vi "8. CoffeeMaker Store and Read Data.vi"() -> ()   [LabVIEW 2018]
doc: "Coffee Machine Version 1.0: store and read non-volatile data of coffee units and brewing chamber operations"
uses:
  Controls/States.ctl
  <vilib>/Utility/miscctls.llb/LVMinMaxIncTypeDef.ctl
  <vilib>/Utility/file.llb/Read Delimited Spreadsheet (DBL).vi
  <vilib>/Utility/file.llb/Read Delimited Spreadsheet (string).vi
  <vilib>/Utility/file.llb/Write Delimited Spreadsheet (DBL).vi
panel:
  out "s? t:f":enum16{"next state", "current state"}(ring)
  out "error out":errorcluster
  in  "error in (no error)":errorcluster
  in  "Power Switch":bool
  in  "Simulation":cluster{"Water":dbl, "Coffee":dbl, "Milk":dbl} caption="Wasser" {"Milk" scale=0.0..100.0; "Water" scale=0.0..100.0; "Coffee" scale=0.0..100.0}
  out "Display":T1 {"Coffee" scale=0.0..80.0; "Brewing Chamber" scale=0.0..80.0}
  in  "Coffee Selection":T2 caption="Selection" {"Type" min=0 max=2 step=1 scale=0.0..2.0}
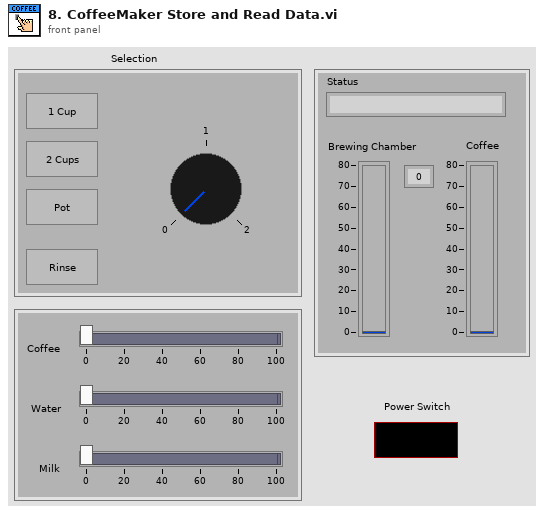
[diagram p1: front panel]
types:
  T1 = cluster{"Brewing Chamber":dbl, "Coffee":dbl, "Status":string, "Remaining Time:":i32}
  T2 = cluster{"1 Cup":bool, "2 Cups":bool, "Pot":bool, "Rinse":bool, "Type":i8}
  T3 = cluster{"Status":refnum<vi>, "Brewing Chamber":refnum<vi>, "Coffee":refnum<vi>, "Power Switch":refnum<vi>}
  T4 = enum8{"Enabled", "Disabled", "Disabled and Grayed Out"}
  T5 = typedef "LVMinMaxIncTypeDef.ctl" = cluster{"Minimum":dbl, "Maximum":dbl, "Increment":dbl}
  T6 = typedef "States.ctl" = enum16{"Initialize", "Set Language", "Wait for Power On", "Heat up", "Check and Wait for Water", "Rinsing", "Check Resources", "User Input", "Grinding", "Boiling", "Pouring", "Rinse before Stop", "Write Data", "Stop"}
  T7 = cluster{"Coffee":refnum<vi>, "Water":refnum<vi>, "Milk":refnum<vi>}
  T8 = cluster{"Coffee Selection":refnum<vi>, "1 Cup":refnum<vi>, "2 Cups":refnum<vi>, "Pot":refnum<vi>, "Rinse":refnum<vi>, "Type":refnum<vi>}
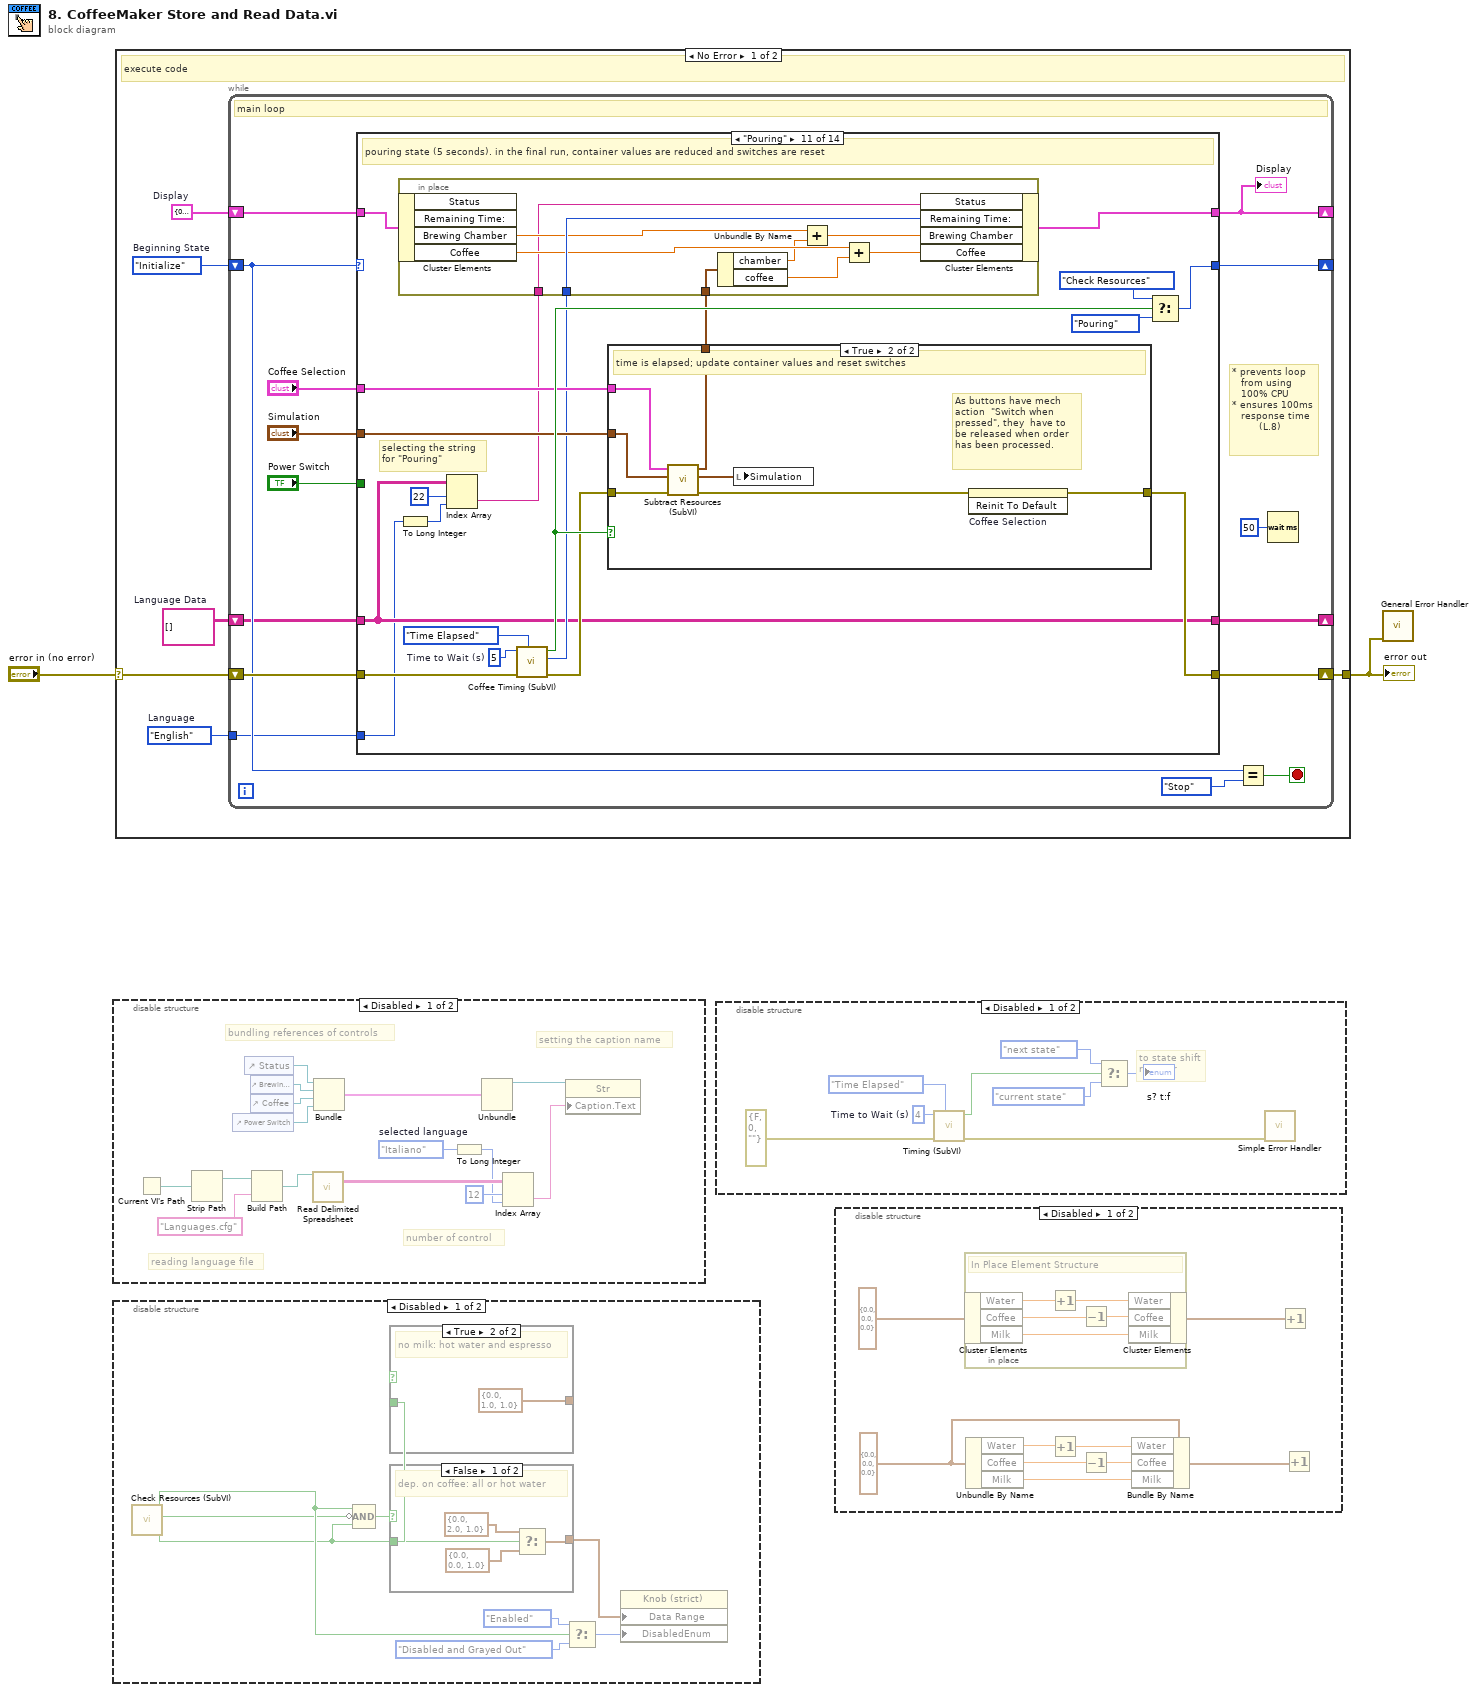
[diagram p0: block diagram]
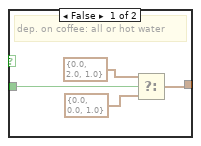
[diagram p3: hidden frame]
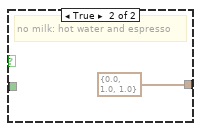
[diagram p4: hidden frame]
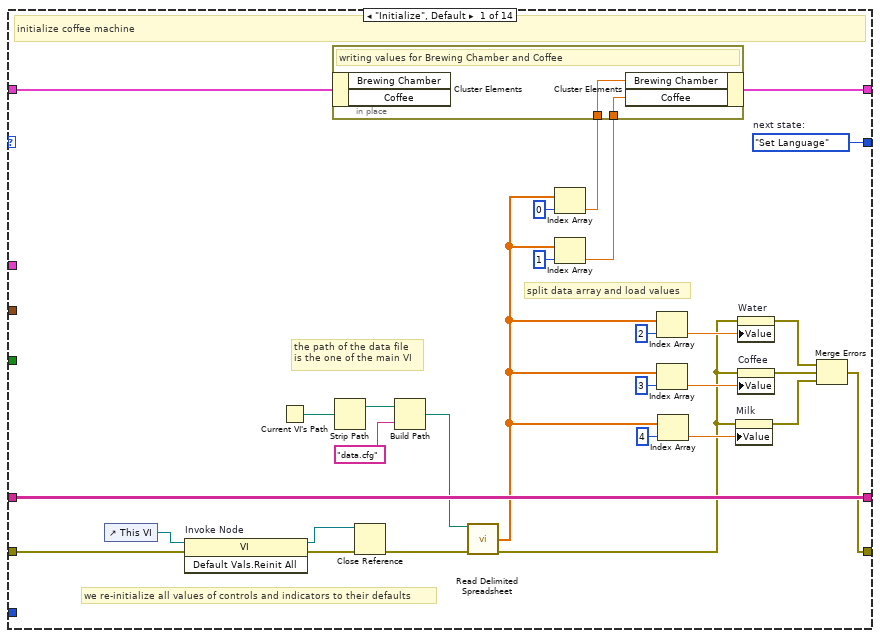
[diagram p8: hidden frame]
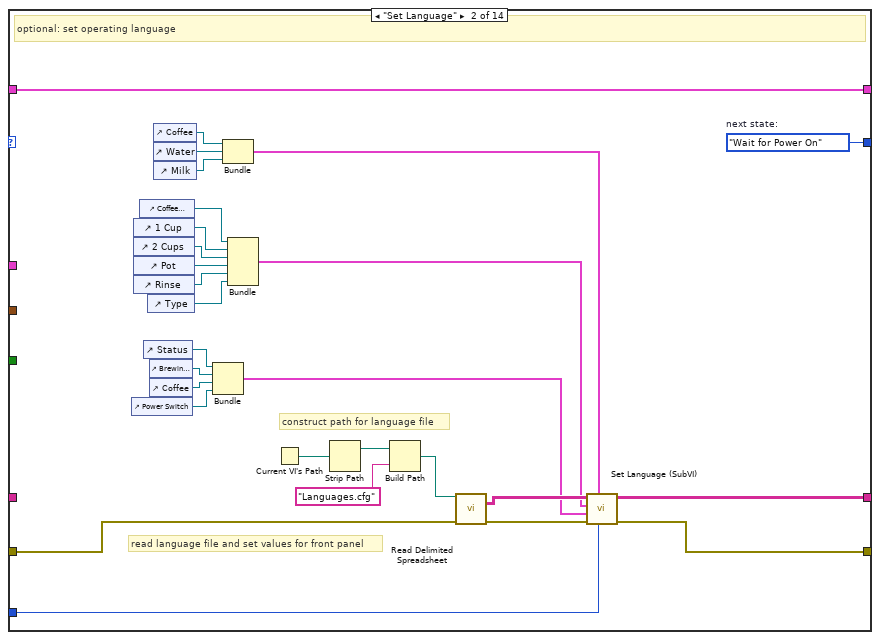
[diagram p9: hidden frame]
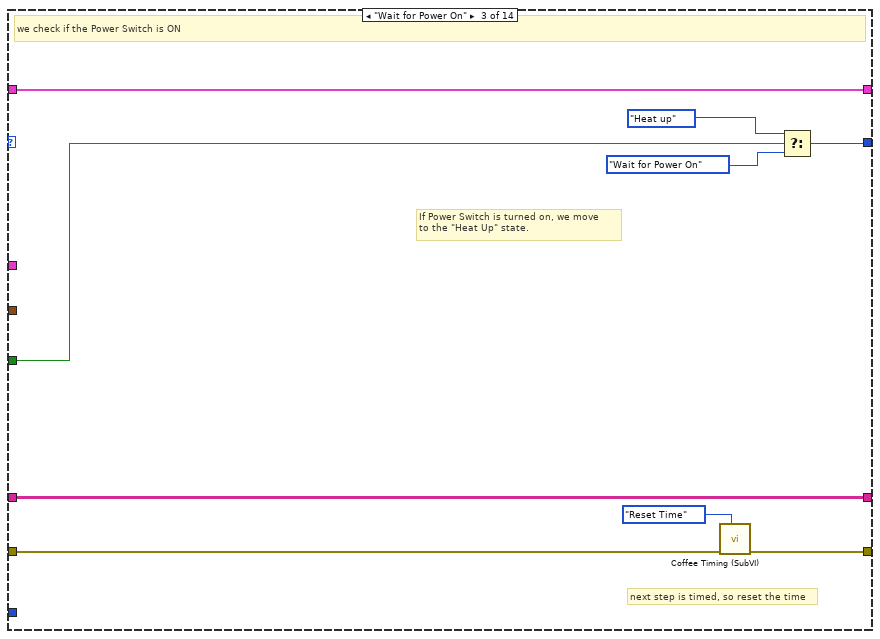
[diagram p10: hidden frame]
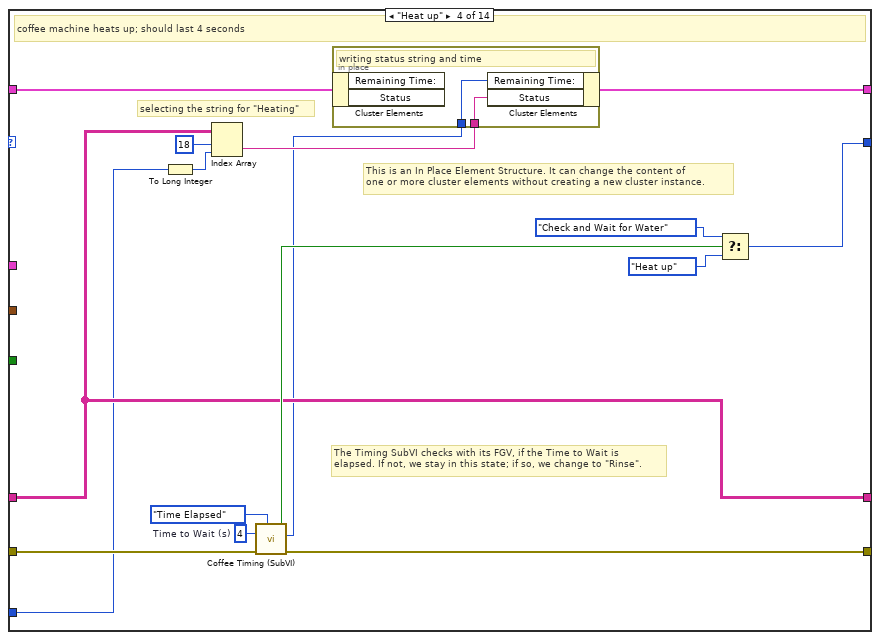
[diagram p11: hidden frame]
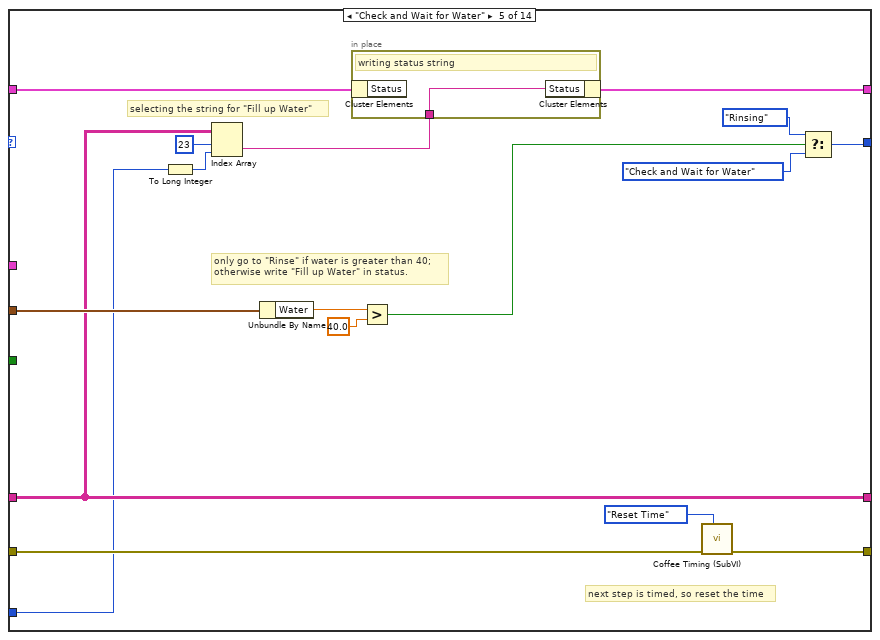
[diagram p12: hidden frame]
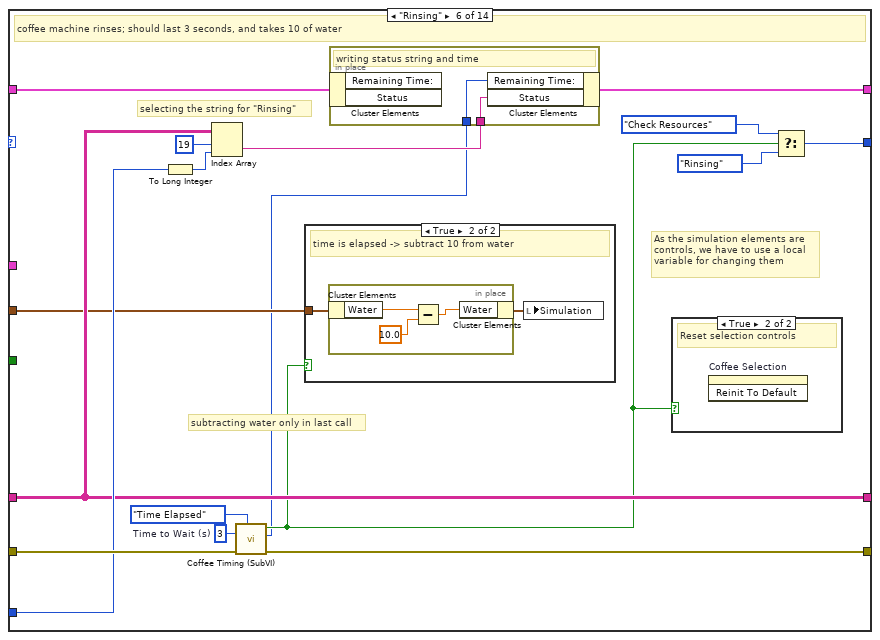
[diagram p13: hidden frame]
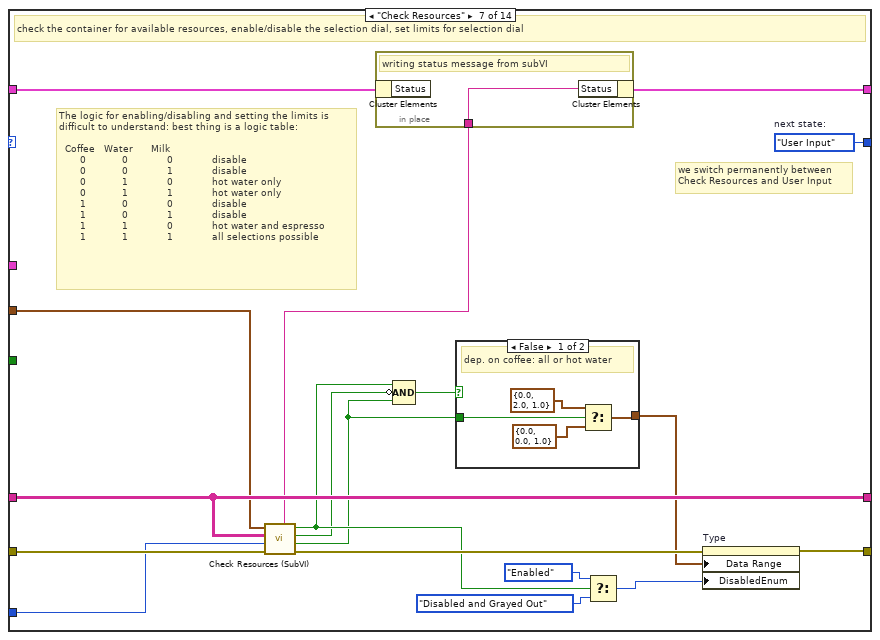
[diagram p16: hidden frame]
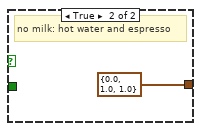
[diagram p17: hidden frame]
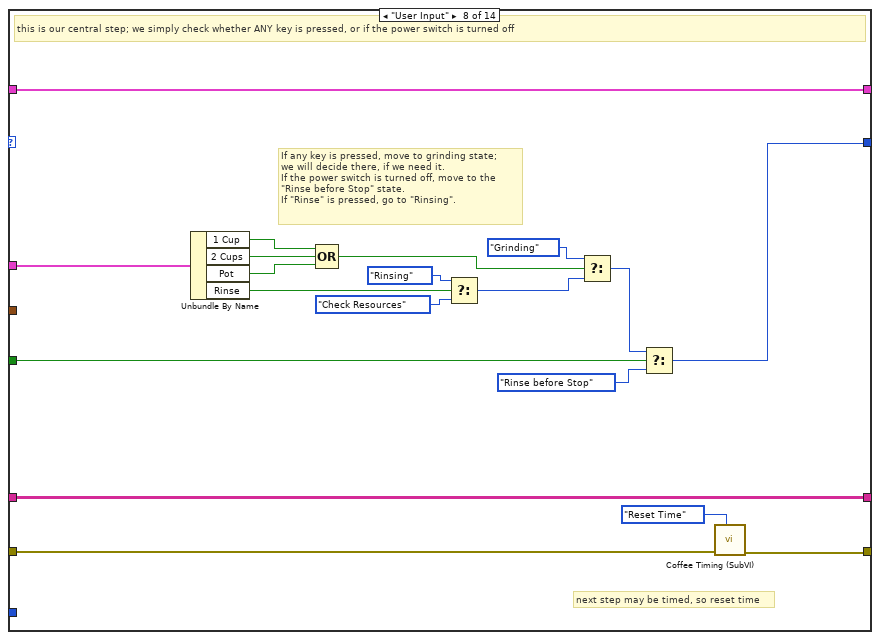
[diagram p18: hidden frame]
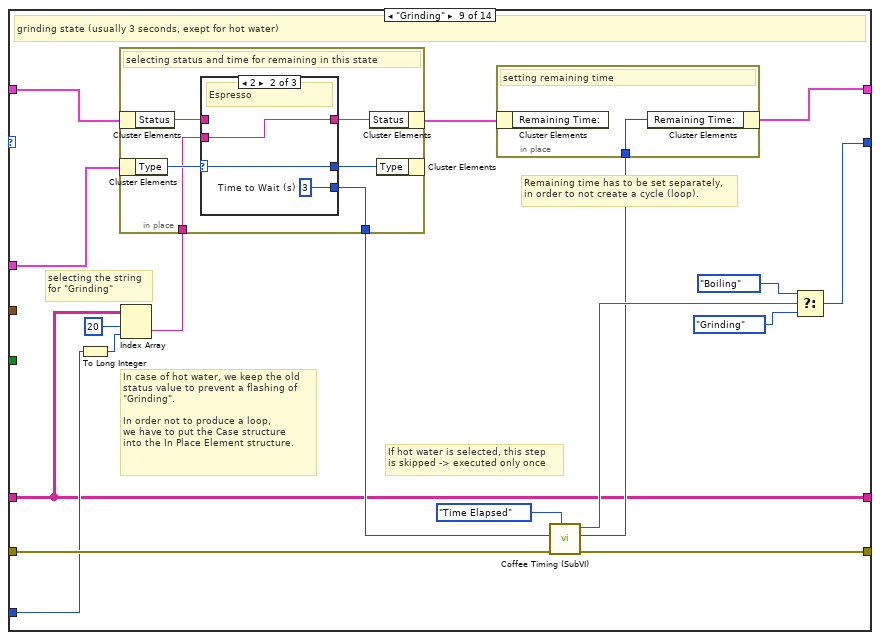
[diagram p19: hidden frame]
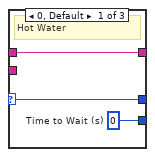
[diagram p20: hidden frame]
diagram:
  n1 = disable-structure shown="Disabled" {
    frame Disabled {
      w5 = enum16{"English", "Deutsch", "Italiano"}."Italiano"  # selected language
      # "setting the caption name"
      # "number of control"
      # "reading language file"
      # "bundling references of controls"
      n2 = Current VI's Path() -> (path=w11:path)
      n3 = Strip Path(path=w11) -> (stripped path=w10:path)  [unwired: 1 out]
      n4 = control-ref of="Power Switch"() -> (w17:refnum<vi>)
      n5 = control-ref of="Status"() -> (w14:refnum<vi>)
      n6 = control-ref of="Brewing Chamber"() -> (w15:refnum<vi>)
      n7 = control-ref of="Coffee"() -> (w16:refnum<vi>)
      n8 = Build Path(base path=w10, name or relative path="Languages.cfg") -> (appended path=w8:path)
      n9 = call-poly <vilib>:"Read Delimited Spreadsheet.vi"("file path (dialog if empty)"=w8) -> ("all rows"=w7:string[][])  [unwired: 9 in, 5 out]
      n10 = Bundle("Status"=w14, "Brewing Chamber"=w15, "Coffee"=w16, "Power Switch"=w17) -> (w13:T3)  [unwired: 1 in]
      n11 = To Long Integer(number=w5) -> (32bit integer=w4:i32)
      n12 = Unbundle(w13) -> ("Status"=w12:refnum<vi>)  [unwired: 3 out]
      n13 = Index Array(array=w7, index (row)=12, index (col)=w4) -> (element=w3:string)
      n14 = property class="Str"(reference=w12, "Caption.Text"=w3) -> ()  [unwired: 1 in, 2 out]
    }
    frame Enabled {
    }
  }
  n15 = disable-structure shown="Disabled" {
    frame Disabled {
      n16 = call "Check Resources (SubVI).vi"() -> ("Coffee ok?"=w18:bool, "Milk ok?"=w19:bool, "Water ok?"=w20:bool)  [unwired: 7 in, 2 out]
      n17 = Compound Arithmetic op=AND(w20, invert w19, w18) -> (w22:bool)
      n18 = case shown="True" {
        selector: _ -> [_ _]
        tunnel: w18 -> [w27 _]
        tunnel: [w26 T5 {"Minimum"=0.0, "Maximum"=1.0, "Increment"=1.0} ("Data Entry Limits")] -> _
        frame False {
          # "dep. on coffee: all or hot water"
          n19 = Select(t=T5 {"Minimum"=0.0, "Maximum"=2.0, "Increment"=1.0} ("Data Entry Limits"), s=w27, f=T5 {"Minimum"=0.0, "Maximum"=0.0, "Increment"=1.0} ("Data Entry Limits")) -> (s? t:f=w26:T5)
        }
        frame True {
          # "no milk: hot water and espresso"
        }
      }
      n20 = case shown="False" w22 {
        tunnel: w18 -> [w32 _]
        tunnel: [w31 T5 {"Minimum"=0.0, "Maximum"=1.0, "Increment"=1.0} ("Data Entry Limits")] -> w21
        frame False {
          # "dep. on coffee: all or hot water"
          n21 = Select(t=T5 {"Minimum"=0.0, "Maximum"=2.0, "Increment"=1.0} ("Data Entry Limits"), s=w32, f=T5 {"Minimum"=0.0, "Maximum"=0.0, "Increment"=1.0} ("Data Entry Limits")) -> (s? t:f=w31:T5)
        }
        frame True {
          # "no milk: hot water and espresso"
        }
      }
      n22 = Select(t=T4."Enabled" ("Disabled"), s=w20, f=T4."Disabled and Grayed Out" ("Disabled")) -> (s? t:f=w23:T4)
      n23 = property on="Property Node" class="Knob (strict)"("Data Range"=w21, "DisabledEnum"=w23) -> ()  [unwired: 2 in, 2 out]
    }
    frame Enabled {
    }
  }
  n24 = case shown="No Error" "error in (no error)" {
    selector: "error in (no error)" -> [w40 w365]
    tunnel: [w41 w365] -> w1
    frame No Error {
      w36 = T1 {"Brewing Chamber"=0.0, "Coffee"=0.0, "Status"="", "Remaining Time:"=0}  # Display
      w37 = enum16{"English", "Deutsch", "Italiano"}."English"  # Language
      w38 = string[][] []  # Language Data
      w39 = States."Initialize"  # Beginning State
      # "execute code"
      n25 = while {
        shift-right: [w53] -> _
        shift-left: w39 -> [w52]
        shift-right: [w46] -> _
        shift-left: w38 -> [w45]
        shift-right: [w42] -> _
        shift-left: w36 -> [w49]
        shift-right: [w56] -> w41
        shift-left: w40 -> [w55]
        tunnel: w37 -> [w43]
        stop <- w50 stop-if-true
        # "* prevents loop\n   from using\n   100% CPU\n* ensures 100ms\n   response time\n         (L.8)"
        # "main loop"
        n26 = case shown="\"Pouring\"" w52 {
          tunnel: [w74 w108 w119 w139 w150 w176 w192 w225 w243 w274 w287 w334 w353 w361] -> w56
          tunnel: w55 -> [w85 w109 w120 w140 w151 w177 w202 w226 w244 w275 w297 w335 w354 w361]
          tunnel: "Power Switch" -> [_ _ w124 _ _ _ _ w223 _ _ _ _ _ _]
          tunnel: [w84 w106 w123 w136 w157 w173 w196 w222 w240 w270 w294 w331 States."Stop" ("f") States."Stop" ("f")] -> w53
          tunnel: [w63 w105 w117 w131 w143 w169 w197 w213 w233 w276 w298 w328 w351 w363] -> w42
          tunnel: w49 -> [w64 w105 w117 w132 w149 w170 w199 w213 w245 w277 w299 w329 w351 w363]
          tunnel: "Coffee Selection" -> [_ _ _ _ _ _ _ w221 w237 _ w289 _ _ _]
          tunnel: "Simulation" -> [_ _ _ _ w156 w163 w200 _ _ _ w290 w323 w352 _]
          tunnel: [w83 w107 w116 w130 w146 w165 w201 w227 w229 w264 w282 w324 w359 w362] -> w46
          tunnel: w45 -> [w83 _ w116 w130 w146 w165 w201 w227 w229 w264 w282 w324 w359 w362]
          tunnel: w43 -> [_ w92 _ w127 w145 w166 w185 _ w230 w263 w281 w325 _ _]
          frame "Initialize", Default {
            w84 = States."Set Language"  # next state:
            # "split data array and load values"
            # "the path of the data file \nis the one of the main VI"
            # "we re-initialize all values of controls and indicators to their defaults"
            # "initialize coffee machine"
            n27 = control-ref of="This VI"() -> (w59:refnum<vi>)
            n28 = invoke on="Invoke Node" class="VI" method="Default Vals.Reinit All"(reference=w59, error in=w85) -> (reference out=w58:refnum<vi>, error out=w57:errorcluster)  [unwired: 1 in, 1 out]
            n29 = Current VI's Path() -> (path=w81:path)
            n30 = Strip Path(path=w81) -> (stripped path=w80:path)  [unwired: 1 out]
            n31 = Close Reference(reference=w58, error in (no error)=w57) -> (error out=w82:errorcluster)
            n32 = Build Path(base path=w80, name or relative path="data.cfg") -> (appended path=w78:path)
            n33 = call-poly <vilib>:"Read Delimited Spreadsheet.vi"("file path (dialog if empty)"=w78, "error in (no error)"=w82) -> ("first row"=w77:dbl[], "error out"=w60:errorcluster)  [unwired: 8 in, 4 out]
            n34 = Index Array "Index Array"(array=w77, index=0) -> (element=w62:dbl)
            n35 = Index Array(array=w77, index=1) -> (element=w61:dbl)
            n36 = in-place {
              in-place-border: w62 -> [w87]
              in-place-border: w61 -> [w86]
              # "writing values for Brewing Chamber and Coffee"
              n37 = in-place-cluster #1(w64) -> ()  [unwired: 2 out]
              n38 = in-place-cluster #1("Brewing Chamber"=w87, "Coffee"=w86) -> (w63:T1)
            }
            n39 = Index Array(array=w77, index=2) -> (element=w68:dbl)
            n40 = Index Array(array=w77, index=3) -> (element=w66:dbl)
            n41 = Index Array(array=w77, index=4) -> (element=w76:dbl)
            n42 = property on="Milk" class="Slide (strict)"(error in=w60, "Value"=w76) -> (error out=w75:errorcluster)  [unwired: 1 in, 1 out]
            n43 = property on="Water" class="Slide (strict)"(error in=w60, "Value"=w68) -> (error out=w67:errorcluster)  [unwired: 1 in, 1 out]
            n44 = property on="Coffee" class="Slide (strict)"(error in=w60, "Value"=w66) -> (error out=w65:errorcluster)  [unwired: 1 in, 1 out]
            n45 = Merge Errors(w67, w65, w75) -> (w74:errorcluster)
          }
          frame "Set Language" {
            w106 = States."Wait for Power On"  # next state:
            # "construct path for language file"
            # "read language file and set values for front panel"
            # "optional: set operating language"
            n46 = control-ref of="Power Switch"() -> (w95:refnum<vi>)
            n47 = control-ref of="1 Cup"() -> (w103:refnum<vi>)
            n48 = control-ref of="2 Cups"() -> (w102:refnum<vi>)
            n49 = control-ref of="Pot"() -> (w101:refnum<vi>)
            n50 = control-ref of="Rinse"() -> (w100:refnum<vi>)
            n51 = control-ref of="Coffee Selection"() -> (w104:refnum<vi>)
            n52 = control-ref of="Status"() -> (w98:refnum<vi>)
            n53 = control-ref of="Type"() -> (w99:refnum<vi>)
            n54 = control-ref of="Brewing Chamber"() -> (w97:refnum<vi>)
            n55 = control-ref of="Coffee"() -> (w96:refnum<vi>)
            n56 = control-ref of="Coffee"() -> (w91:refnum<vi>)
            n57 = control-ref of="Water"() -> (w90:refnum<vi>)
            n58 = control-ref of="Milk"() -> (w89:refnum<vi>)
            n59 = Bundle("Status"=w98, "Brewing Chamber"=w97, "Coffee"=w96, "Power Switch"=w95) -> (w93:T3)  [unwired: 1 in]
            n60 = Bundle("Coffee"=w91, "Water"=w90, "Milk"=w89) -> (w88:T7)  [unwired: 1 in]
            n61 = Bundle("Coffee Selection"=w104, "1 Cup"=w103, "2 Cups"=w102, "Pot"=w101, "Rinse"=w100, "Type"=w99) -> (w94:T8)  [unwired: 1 in]
            n62 = Current VI's Path() -> (path=w110:path)
            n63 = Strip Path(path=w110) -> (stripped path=w111:path)  [unwired: 1 out]
            n64 = Build Path(base path=w111, name or relative path="Languages.cfg") -> (appended path=w113:path)
            n65 = call-poly <vilib>:"Read Delimited Spreadsheet.vi"("file path (dialog if empty)"=w113, "error in (no error)"=w109) -> ("all rows"=w115:string[][], "error out"=w114:errorcluster)  [unwired: 8 in, 4 out]
            n66 = call "Set Language (SubVI).vi"("Language (English)"=w92, "Simulation \nReferences"=w88, "error in (no error)"=w114, "Status\nReferences"=w93, "Selection \nReferences"=w94, "Language Data"=w115) -> ("error out"=w108:errorcluster, "Language Data Out"=w107:string[][])  [unwired: 4 in]
          }
          frame "Wait for Power On" {
            # "next step is timed, so reset the time"
            # "If Power Switch is turned on, we move\nto the \"Heat Up\" state."
            # "we check if the Power Switch is ON"
            n67 = call "Coffee Timing (SubVI).vi"("Function"=enum16{"Reset Time", "Time Elapsed"}."Reset Time", "error in (no error)"=w120) -> ("error out"=w119:errorcluster)  [unwired: 7 in, 2 out]
            n68 = Select(t=States."Heat up" ("Beginning State"), s=w124, f=States."Wait for Power On") -> (s? t:f=w123:T6)
          }
          frame "Heat up" {
            w137 = 4  # Time to Wait (s)
            # "selecting the string for \"Heating\""
            # "This is an In Place Element Structure. It can change the content of\none or more cluster elements without creating a new cluster instance."
            # "The Timing SubVI checks with its FGV, if the Time to Wait is\nelapsed. If not, we stay in this state; if so, we change to \"Rinse\"."
            # "coffee machine heats up; should last 4 seconds"
            n69 = To Long Integer(number=w127) -> (32bit integer=w128:i32)
            n70 = Index Array "Index Array"(array=w130, index (row)=18, index (col)=w128) -> (element=w126:string)
            n71 = call "Coffee Timing (SubVI).vi"("Function"=enum16{"Reset Time", "Time Elapsed"}."Time Elapsed", "error in (no error)"=w140, "Time to Wait (s)"=w137) -> ("error out"=w139:errorcluster, "Remaining Time"=w125:i32, "Time elapsed ?"=w133:bool)  [unwired: 6 in]
            n72 = in-place {
              in-place-border: w126 -> [w142]
              in-place-border: w125 -> [w141]
              # "writing status string and time"
              n73 = in-place-cluster #2(w132) -> ()  [unwired: 2 out]
              n74 = in-place-cluster #2("Remaining Time:"=w141, "Status"=w142) -> (w131:T1)
            }
            n75 = Select(t=States."Check and Wait for Water" ("Beginning State"), s=w133, f=States."Heat up" ("Beginning State")) -> (s? t:f=w136:T6)
          }
          frame "Check and Wait for Water" {
            # "next step is timed, so reset the time"
            # "only go to \"Rinse\" if water is greater than 40;\notherwise write \"Fill up Water\" in status."
            # "selecting the string for \"Fill up Water\""
            n76 = To Long Integer(number=w145) -> (32bit integer=w147:i32)
            n77 = Index Array "Index Array"(array=w146, index (row)=23, index (col)=w147) -> (element=w144:string)
            n78 = Unbundle By Name(w156) -> ("Water"=w155:dbl)
            n79 = in-place {
              in-place-border: w144 -> [w160]
              # "writing status string"
              n80 = in-place-cluster #3(w149) -> ()  [unwired: 1 out]
              n81 = in-place-cluster #3("Status"=w160) -> (w143:T1)
            }
            n82 = Greater?(x=w155, y=40.0) -> (0:w153:bool)
            n83 = call "Coffee Timing (SubVI).vi"("Function"=enum16{"Reset Time", "Time Elapsed"}."Reset Time", "error in (no error)"=w151) -> ("error out"=w150:errorcluster)  [unwired: 7 in, 2 out]
            n84 = Select(t=States."Rinsing" ("f"), s=w153, f=States."Check and Wait for Water") -> (s? t:f=w157:T6)
          }
          frame "Rinsing" {
            w174 = 3  # Time to Wait (s)
            # "subtracting water only in last call"
            # "As the simulation elements are\ncontrols, we have to use a local\nvariable for changing them"
            # "selecting the string for \"Rinsing\""
            # "coffee machine rinses; should last 3 seconds, and takes 10 of water"
            n85 = To Long Integer(number=w166) -> (32bit integer=w167:i32)
            n86 = Index Array "Index Array"(array=w165, index (row)=19, index (col)=w167) -> (element=w164:string)
            n87 = call "Coffee Timing (SubVI).vi"("Function"=enum16{"Reset Time", "Time Elapsed"}."Time Elapsed", "error in (no error)"=w177, "Time to Wait (s)"=w174) -> ("error out"=w176:errorcluster, "Remaining Time"=w161:i32, "Time elapsed ?"=w162:bool)  [unwired: 6 in]
            n88 = case shown="True" w162 {
              tunnel: w163 -> [_ w179]
              frame False {
                # "time is running ..."
              }
              frame True {
                # "time is elapsed -> subtract 10 from water"
                n89 = in-place {
                  n90 = in-place-cluster #4(w179) -> ("Water"=w182:dbl)
                  n91 = Subtract(x=w182, y=10.0) -> (x-y=w180:dbl)
                  n92 = in-place-cluster #4("Water"=w180) -> (w178:cluster{"Water":dbl, "Coffee":dbl, "Milk":dbl})
                }
                n93 = local write "Simulation"(w178) -> ()
              }
            }
            n94 = in-place {
              in-place-border: w164 -> [w184]
              in-place-border: w161 -> [w183]
              # "writing status string and time"
              n95 = in-place-cluster #5(w170) -> ()  [unwired: 2 out]
              n96 = in-place-cluster #5("Remaining Time:"=w183, "Status"=w184) -> (w169:T1)
            }
            n97 = case shown="True" w162 {
              frame False {
              }
              frame True {
                # "Reset selection controls"
                n98 = invoke on="Coffee Selection" class="Clust (strict)" method="Reinit To Default"() -> ()  [unwired: 3 in, 3 out]
              }
            }
            n99 = Select(t=States."Check Resources" ("Beginning State"), s=w162, f=States."Rinsing" ("Beginning State")) -> (s? t:f=w173:T6)
          }
          frame "Check Resources" {
            w196 = States."User Input"  # next state:
            # "The logic for enabling/disabling and setting the limits is \ndifficult to understand: best thing is a logic table:\n\n  Coffee   Water      Milk\n       0            0             0             disable\n       0            0             1             disable\n       0            1             0             hot water only\n       0            1             1             hot water only\n       1            0             0             disable\n       1            0             1             disable\n       1            1             0             hot water and espresso\n       1            1             1             all selections possible"
            # "we switch permanently between \nCheck Resources and User Input"
            # "check the container for available resources, enable/disable the selection dial, set limits for selection dial"
            n100 = call "Check Resources (SubVI).vi"("error in (no error)"=w202, "Language"=w185, "Language Data"=w201, "Simulation"=w200) -> ("error out"=w193:errorcluster, "Coffee ok?"=w187:bool, "Milk ok?"=w189:bool, "Water ok?"=w190:bool, "Status Message"=w198:string)  [unwired: 3 in]
            n101 = in-place {
              in-place-border: w198 -> [w208]
              # "writing status message from subVI"
              n102 = in-place-cluster #6(w199) -> ()  [unwired: 1 out]
              n103 = in-place-cluster #6("Status"=w208) -> (w197:T1)
            }
            n104 = Compound Arithmetic op=AND(w190, invert w189, w187) -> (w188:bool)
            n105 = case shown="False" w188 {
              tunnel: w187 -> [w204 _]
              tunnel: [w203 T5 {"Minimum"=0.0, "Maximum"=1.0, "Increment"=1.0} ("Data Entry Limits")] -> w186
              frame False {
                # "dep. on coffee: all or hot water"
                n106 = Select(t=T5 {"Minimum"=0.0, "Maximum"=2.0, "Increment"=1.0} ("Data Entry Limits"), s=w204, f=T5 {"Minimum"=0.0, "Maximum"=0.0, "Increment"=1.0} ("Data Entry Limits")) -> (s? t:f=w203:T5)
              }
              frame True {
                # "no milk: hot water and espresso"
              }
            }
            n107 = Select(t=T4."Enabled" ("Disabled"), s=w190, f=T4."Disabled and Grayed Out" ("Disabled")) -> (s? t:f=w191:T4)
            n108 = property on="Type" class="Knob (strict)"(error in=w193, "Data Range"=w186, "DisabledEnum"=w191) -> (error out=w192:errorcluster)  [unwired: 1 in, 1 out]
          }
          frame "User Input" {
            # "If any key is pressed, move to grinding state; \nwe will decide there, if we need it.\nIf the power switch is turned off, move to the \n\"Rinse before Stop\" state.\nIf \"Rinse\" is pressed, go to \"Rinsing\"."
            # "next step may be timed, so reset time"
            # "this is our central step; we simply check whether ANY key is pressed, or if the power switch is turned off"
            n109 = Unbundle By Name(w221) -> ("1 Cup"=w220:bool, "2 Cups"=w219:bool, "Pot"=w218:bool, "Rinse"=w212:bool)
            n110 = Compound Arithmetic op=OR(w220, w219, w218) -> (w215:bool)
            n111 = Select(t=States."Rinsing", s=w212, f=States."Check Resources" ("t")) -> (s? t:f=w209:T6)
            n112 = Select(t=States."Grinding", s=w215, f=w209) -> (s? t:f=w216:T6)
            n113 = Select(t=w216, s=w223, f=States."Rinse before Stop") -> (s? t:f=w222:T6)
            n114 = call "Coffee Timing (SubVI).vi"("Function"=enum16{"Reset Time", "Time Elapsed"}."Reset Time", "error in (no error)"=w226) -> ("error out"=w225:errorcluster)  [unwired: 7 in, 2 out]
          }
          frame "Grinding" {
            # "selecting the string \nfor \"Grinding\""
            # "Remaining time has to be set separately,\nin order to not create a cycle (loop)."
            # "In case of hot water, we keep the old\nstatus value to prevent a flashing of\n\"Grinding\".\n\nIn order not to produce a loop,\nwe have to put the Case structure\ninto the In Place Element structure."
            # "If hot water is selected, this step\nis skipped -> executed only once"
            # "grinding state (usually 3 seconds, exept for hot water)"
            n115 = To Long Integer(number=w230) -> (32bit integer=w231:i32)
            n116 = Index Array "Index Array"(array=w229, index (row)=20, index (col)=w231) -> (element=w228:string)
            n117 = in-place {
              in-place-border: [w249] -> w236
              in-place-border: w228 -> [w247]
              # "selecting status and time for remaining in this state"
              n118 = in-place-cluster #7(w245) -> ("Status"=w251:string)
              n119 = in-place-cluster #8(w237) -> ("Type"=w252:i8)
              n120 = case shown="2" w252 {
                selector: w252 -> [w253 w257 w260]
                tunnel: [w255 w258 w261] -> w249
                tunnel: [w254 w256 w259] -> w250
                tunnel: w251 -> [w254 _ _]
                tunnel: [w253 w257 w260] -> w248
                tunnel: w247 -> [_ w256 w259]
                frame 0, Default {
                  w255 = 0  # Time to Wait (s)
                  # "Hot Water"
                }
                frame 2 {
                  w258 = 3  # Time to Wait (s)
                  # "Espresso"
                }
                frame 1 {
                  w261 = 3  # Time to Wait (s)
                  # "Coffee"
                }
              }
              n121 = in-place-cluster #7("Status"=w250) -> (w235:T1)
              n122 = in-place-cluster #8("Type"=w248) -> ()  [unwired: 1 out]
            }
            n123 = call "Coffee Timing (SubVI).vi"("Function"=enum16{"Reset Time", "Time Elapsed"}."Time Elapsed", "error in (no error)"=w244, "Time to Wait (s)"=w236) -> ("error out"=w243:errorcluster, "Remaining Time"=w234:i32, "Time elapsed ?"=w241:bool)  [unwired: 6 in]
            n124 = in-place {
              in-place-border: w234 -> [w246]
              # "setting remaining time"
              n125 = in-place-cluster #9(w235) -> ()  [unwired: 1 out]
              n126 = in-place-cluster #9("Remaining Time:"=w246) -> (w233:T1)
            }
            n127 = Select(t=States."Boiling" ("Beginning State"), s=w241, f=States."Grinding") -> (s? t:f=w240:T6)
          }
          frame "Boiling" {
            w273 = 3  # Time to Wait (s)
            # "selecting the string for \"Boiling\""
            # "nothing special happens here"
            # "boiling state (3 seconds)"
            n128 = To Long Integer(number=w263) -> (32bit integer=w265:i32)
            n129 = Index Array "Index Array"(array=w264, index (row)=19, index (col)=w265) -> (element=w262:string)
            n130 = call "Coffee Timing (SubVI).vi"("Function"=enum16{"Reset Time", "Time Elapsed"}."Time Elapsed", "error in (no error)"=w275, "Time to Wait (s)"=w273) -> ("error out"=w274:errorcluster, "Remaining Time"=w267:i32, "Time elapsed ?"=w271:bool)  [unwired: 6 in]
            n131 = in-place {
              in-place-border: w267 -> [w279]
              in-place-border: w262 -> [w278]
              n132 = in-place-cluster #10(w277) -> ()  [unwired: 2 out]
              n133 = in-place-cluster #10("Status"=w278, "Remaining Time:"=w279) -> (w276:T1)
            }
            n134 = Select(t=States."Pouring" ("Beginning State"), s=w271, f=States."Boiling") -> (s? t:f=w270:T6)
          }
          frame "Pouring" {
            w296 = 5  # Time to Wait (s)
            # "selecting the string \nfor \"Pouring\""
            # "pouring state (5 seconds). in the final run, container values are reduced and switches are reset"
            n135 = To Long Integer(number=w281) -> (32bit integer=w283:i32)
            n136 = Index Array "Index Array"(array=w282, index (row)=22, index (col)=w283) -> (element=w280:string)
            n137 = call "Coffee Timing (SubVI).vi"("Function"=enum16{"Reset Time", "Time Elapsed"}."Time Elapsed", "error in (no error)"=w297, "Time to Wait (s)"=w296) -> ("error out"=w288:errorcluster, "Remaining Time"=w286:i32, "Time elapsed ?"=w291:bool)  [unwired: 6 in]
            n138 = case shown="True" w291 {
              tunnel: w290 -> [_ w307]
              tunnel: w289 -> [_ w308]
              tunnel: w288 -> [w301 w305]
              tunnel: [w301 w303] -> w287
              tunnel: [cluster{"coffee":dbl, "chamber":dbl} {"coffee"=0.0, "chamber"=0.0} ("Coffe and Chamber increase") w302] -> w285
              frame False {
                # "... time is still running ..."
              }
              frame True {
                # "As buttons have mech \naction  \"Switch when \npressed\", they  have to \nbe released when order \nhas been processed."
                # "time is elapsed; update container values and reset switches"
                n139 = call "Subtract Resources (SubVI).vi"("error in (no error)"=w305, "Simulation in"=w307, "Coffee Selection"=w308) -> ("error out"=w304:errorcluster, "Simulation out"=w306:cluster{"Water":dbl, "Coffee":dbl, "Milk":dbl}, "Coffe and Chamber increase"=w302:cluster{"coffee":i8, "chamber":i8})  [unwired: 6 in]
                n140 = local write "Simulation"(w306) -> ()
                n141 = invoke on="Coffee Selection" class="Clust (strict)" method="Reinit To Default"(error in=w304) -> (error out=w303:errorcluster)  [unwired: 2 in, 2 out]
              }
            }
            n142 = in-place {
              in-place-border: w286 -> [w317]
              in-place-border: w285 -> [w316]
              in-place-border: w280 -> [w309]
              n143 = in-place-cluster #11(w299) -> ("Brewing Chamber"=w315:dbl, "Coffee"=w313:dbl)  [unwired: 2 out]
              n144 = Unbundle By Name(w316) -> ("chamber"=w310:dbl, "coffee"=w311:dbl)
              n145 = Add(x=w315, y=w310) -> (x+y=w314:dbl)
              n146 = Add(x=w313, y=w311) -> (x+y=w312:dbl)
              n147 = in-place-cluster #11("Status"=w309, "Remaining Time:"=w317, "Brewing Chamber"=w314, "Coffee"=w312) -> (w298:T1)
            }
            n148 = Select(t=States."Check Resources" ("Beginning State"), s=w291, f=States."Pouring") -> (s? t:f=w294:T6)
          }
          frame "Rinse before Stop" {
            w332 = 3  # Time to Wait (s)
            # "subtracting water only in last call"
            # "selecting the string for \"Rinsing\""
            # "coffee machine rinses before stopping; should last 3 seconds, and takes 10 of water"
            n149 = To Long Integer(number=w325) -> (32bit integer=w326:i32)
            n150 = Index Array "Index Array"(array=w324, index (row)=19, index (col)=w326) -> (element=w319:string)
            n151 = call "Coffee Timing (SubVI).vi"("Function"=enum16{"Reset Time", "Time Elapsed"}."Time Elapsed", "error in (no error)"=w335, "Time to Wait (s)"=w332) -> ("error out"=w334:errorcluster, "Remaining Time"=w318:i32, "Time elapsed ?"=w321:bool)  [unwired: 6 in]
            n152 = case shown="True" w321 {
              tunnel: [w336 ""] -> w320
              tunnel: w319 -> [w336 _]
              frame False {
                # "write status"
              }
              frame True {
                # "clear status"
              }
            }
            n153 = in-place {
              in-place-border: w320 -> [w344]
              in-place-border: w318 -> [w343]
              # "writing status string"
              n154 = in-place-cluster #12(w329) -> ()  [unwired: 2 out]
              n155 = in-place-cluster #12("Status"=w344, "Remaining Time:"=w343) -> (w328:T1)
            }
            n156 = case shown="True" w321 {
              tunnel: w323 -> [_ w339]
              frame False {
                # "time is running ..."
              }
              frame True {
                # "time is elapsed -> subtract 10 from water"
                n157 = in-place {
                  n158 = in-place-cluster #13(w339) -> ("Water"=w342:dbl)
                  n159 = Subtract(x=w342, y=10.0) -> (x-y=w340:dbl)
                  n160 = in-place-cluster #13("Water"=w340) -> (w338:cluster{"Water":dbl, "Coffee":dbl, "Milk":dbl})
                }
                n161 = local write "Simulation"(w338) -> ()
              }
            }
            n162 = Select(t=States."Write Data" ("Beginning State"), s=w321, f=States."Rinse before Stop") -> (s? t:f=w331:T6)
          }
          frame "Write Data" {
            # "the path of the data file \nis the one of the main VI"
            # "writing the data from the status indicators"
            n163 = Unbundle By Name(w351) -> ("Brewing Chamber"=w350:dbl, "Coffee"=w349:dbl)
            n164 = Unbundle By Name(w352) -> ("Water"=w348:dbl, "Coffee"=w347:dbl, "Milk"=w346:dbl)
            n165 = Build Array(w350, w349, w348, w347, w346) -> (w345:dbl[])
            n166 = Current VI's Path() -> (path=w358:path)
            n167 = Strip Path(path=w358) -> (stripped path=w357:path)  [unwired: 1 out]
            n168 = Build Path(base path=w357, name or relative path="data.cfg") -> (appended path=w355:path)
            n169 = call-poly <vilib>:"Write Delimited Spreadsheet.vi"("file path (dialog if empty)"=w355, "1D data"=w345, "error in (no error)"=w354) -> ("error out"=w353:errorcluster)  [unwired: 11 in, 1 out]
          }
          frame "Stop" {
            # "this one is just to make sure the program stops"
          }
        }
        "Display" <- w42
        n170 = Equal?(x=w52, y=States."Stop") -> (x = y?=w50:bool)
        n171 = Wait (ms)(milliseconds to wait=u32 50) -> ()  [unwired: 1 out]
      }
    }
    frame Error {
      # "do nothing"
    }
  }
  "error out" <- w1
  n172 = disable-structure shown="Disabled" {
    frame Disabled {
      w372 = 4  # Time to Wait (s)
      # "to state shift\nregister"
      n173 = call "Timing (SubVI).vi"("Function"=enum16{"Reset Time", "Time Elapsed"}."Time Elapsed", "error in (no error)"=errorcluster {"status"=FALSE, "code"=0, "source"=""}, "Time to Wait (s)"=w372) -> ("error out"=w370:errorcluster, "Time elapsed ?"=w369:bool)  [unwired: 6 in, 1 out]
      n174 = Select(t=enum16{"next state", "current state"}."next state", s=w369, f=enum16{"next state", "current state"}."current state") -> (s? t:f=→"s? t:f":enum16{"next state", "current state"})
      n175 = call <vilib>:"Simple Error Handler.vi"("error in (no error)"=w370) -> ()  [unwired: 4 in, 5 out]
    }
    frame Enabled {
    }
  }
  n176 = disable-structure shown="Disabled" {
    frame Disabled {
      w380 = cluster{"Water":dbl, "Coffee":dbl, "Milk":dbl} {"Water"=0.0, "Coffee"=0.0, "Milk"=0.0} ("Simulation")
      n177 = in-place {
        # "In Place Element Structure"
        n178 = in-place-cluster #14(cluster{"Water":dbl, "Coffee":dbl, "Milk":dbl} {"Water"=0.0, "Coffee"=0.0, "Milk"=0.0} ("Simulation")) -> ("Water"=w387:dbl, "Coffee"=w385:dbl, "Milk"=w383:dbl)
        n179 = Increment(x=w387) -> (x+1=w386:dbl)
        n180 = Decrement(x=w385) -> (x-1=w384:dbl)
        n181 = in-place-cluster #14("Water"=w386, "Coffee"=w384, "Milk"=w383) -> (w381:cluster{"Water":dbl, "Coffee":dbl, "Milk":dbl})
      }
      n182 = Unbundle By Name(w380) -> ("Water"=w379:dbl, "Coffee"=w376:dbl, "Milk"=w375:dbl)
      n183 = Increment(x=w379) -> (x+1=w378:dbl)
      n184 = Decrement(x=w376) -> (x-1=w377:dbl)
      n185 = Bundle By Name(cluster=w380, "Water"=w378, "Coffee"=w377, "Milk"=w375) -> (w374:cluster{"Water":dbl, "Coffee":dbl, "Milk":dbl})
      n186 = Increment(x=w381) -> ()  [unwired: 1 out]
      n187 = Increment(x=w374) -> ()  [unwired: 1 out]
    }
    frame Enabled {
    }
  }
  n188 = call <vilib>:"General Error Handler.vi"("error in (no error)"=w1) -> ()  [unwired: 10 in, 5 out]
